vi "Emergency Send To Specific Target.vi"(6 "Paras In":variant, 8 "error in (no error)":errorcluster, 9 "Mail Strategy In":refnum<class "Mail Strategy.lvclass">, 10 "Message In":refnum<class "Message.lvclass">, 11 "Map Tree Queue Messenger in":refnum<class "Map Tree Queue Messenger.lvclass">) -> (0 "error out":errorcluster, 3 "Map Tree Queue Messenger out":refnum<class "Map Tree Queue Messenger.lvclass">)   [LabVIEW 2024, in "Map Tree Queue Messenger.lvclass"]
uses:
  Map Tree Queue Messenger.lvclass
  Ancestor Class/Message/Message.lvclass
  Ancestor Class/Messenger/Mail Strategy/Mail Strategy.lvclass
  Mailman/Simple Tree Queue Mailman/Simple Tree Queue Mailman.lvclass
  Ancestor Class/Messenger/Messenger Map Composite/Messenger Map Composite.lvclass/Messenger Map Composite.ctl
  Mailman/Simple Tree Queue Mailman/Simple Tree Queue Mailman.lvclass/Simple Tree Queue Mailman.ctl
  Map Tree Queue Messenger.lvclass/Map Tree Queue Messenger.ctl
  Mailman/Simple Tree Queue Mailman/Public Data/Write Address Recursive Access.vi
  Ancestor Class/Messenger/Messenger Map Composite/Public Data/Read Child Nodes.vi
  Ancestor Class/Messenger/Messenger/Messenger.lvclass
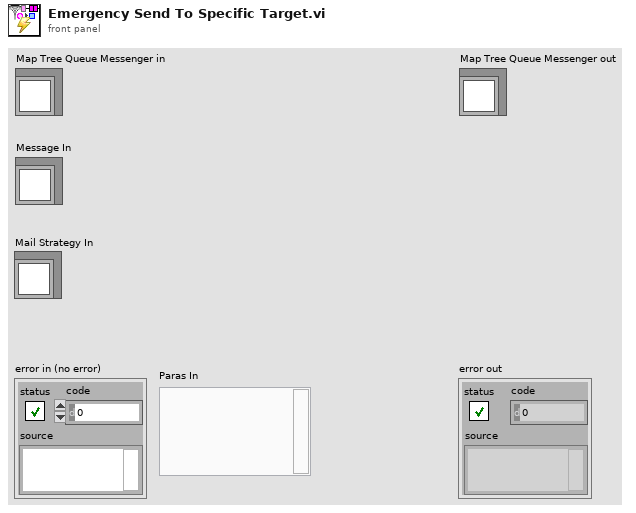
[diagram p1: front panel]
types:
  T1 = typedef "Message Queue.ctl" = refnum<queue>
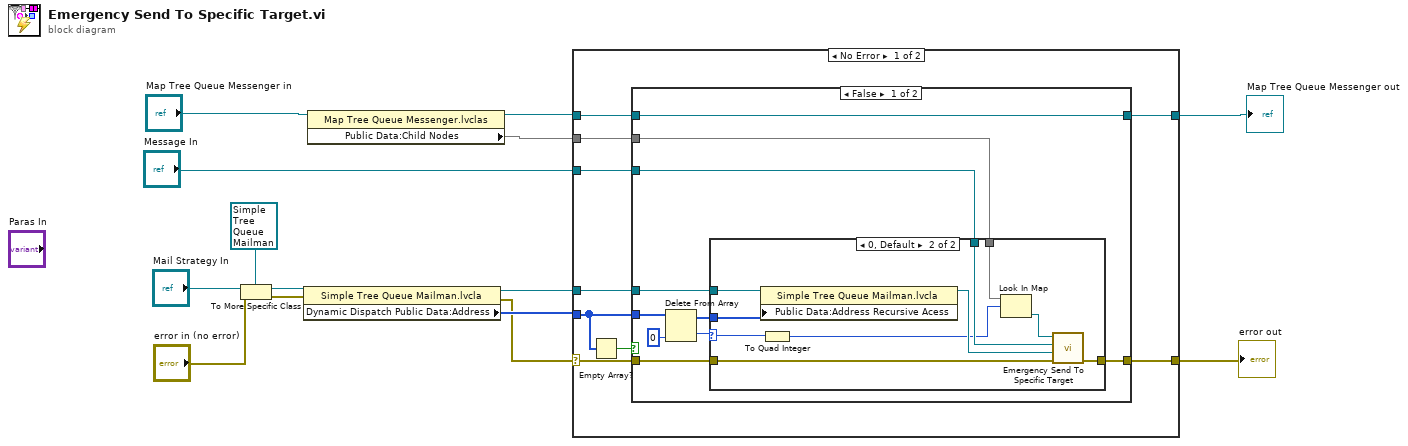
[diagram p0: block diagram]
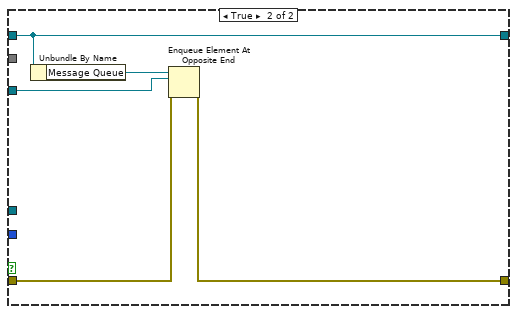
[diagram p3: hidden frame]
diagram:
  n1 = To More Specific Class(target class=refnum<class "Simple Tree Queue Mailman.lvclass"> refnum ("Array Location Mailman.lvclass"), reference="Mail Strategy In", error in="error in (no error)") -> (specific class reference=w12:refnum<class "Simple Tree Queue Mailman.lvclass">, error out=w13:errorcluster)
  n2 = property class="Simple Tree Queue Mailman.lvcla"(reference=w12, error in=w13) -> (reference out=w9:refnum<class "Simple Tree Queue Mailman.lvclass">, error out=w10:errorcluster, "Dynamic Dispatch Public Data:Address"=w11:i32[])
  n3 = property class="Map Tree Queue Messenger.lvclas"(reference="Map Tree Queue Messenger in") -> (reference out=w8:refnum<class "Map Tree Queue Messenger.lvclass">, "Public Data:Child Nodes"=w7:map{i64, refnum<class "Messenger.lvclass">})  [unwired: 1 in, 1 out]
  n4 = case shown="No Error" w10 {
    selector: w10 -> [w18 w50]
    tunnel: w8 -> [w22 w51]
    tunnel: [w20 w51] -> w5
    tunnel: [w17 w50] -> w1
    tunnel: w11 -> [w19 _]
    tunnel: "Message In" -> [w21 _]
    tunnel: w9 -> [w15 _]
    tunnel: w7 -> [w16 _]
    frame No Error {
      n5 = Empty Array?(array=w19) -> (empty?=w23:bool)
      n6 = case shown="False" w23 {
        tunnel: w22 -> [w33 w49]
        tunnel: w21 -> [w30 w47]
        tunnel: [w33 w49] -> w20
        tunnel: w19 -> [w32 _]
        tunnel: w18 -> [w29 w46]
        tunnel: [w28 w45] -> w17
        tunnel: w16 -> [w27 _]
        tunnel: w15 -> [w25 _]
        frame False {
          n7 = Delete From Array(array=w32, index=0) -> (deleted portion=w24:i32, array with subset deleted=w26:i32[])  [unwired: 1 in]
          n8 = case shown="0, Default" w24 {
            selector: w24 -> [_ w36]
            tunnel: w30 -> [_ w44]
            tunnel: w29 -> [w34 w43]
            tunnel: [w34 w42] -> w28
            tunnel: w27 -> [_ w38]
            tunnel: w26 -> [_ w41]
            tunnel: w25 -> [_ w40]
            frame -2147483648..-1 {
            }
            frame 0, Default {
              n9 = property class="Simple Tree Queue Mailman.lvcla"(reference=w40, "Public Data:Address Recursive Acess"=w41) -> (reference out=w39:refnum<class "Simple Tree Queue Mailman.lvclass">)  [unwired: 1 in, 1 out]
              n10 = To Quad Integer(1:w36) -> (0:w35:i64)
              n11 = Look In Map(map=w38, key=w35) -> (value=w37:refnum<class "Messenger.lvclass">)  [unwired: 1 in, 1 out]
              n12 = call-dynamic "Emergency Send To Specific Target.vi"("error in (no error)"=w43, "Mail Strategy In"=w39, "Message In"=w44, "Messenger in"=w37) -> ("error out"=w42:errorcluster)  [unwired: 6 in, 1 out]
            }
          }
        }
        frame True {
          n13 = Unbundle By Name(w49) -> ("Message Queue"=w48:T1)
          n14 = Enqueue Element At Opposite End(queue=w48, element=w47, error in (no error)=w46) -> (error out=w45:errorcluster)  [unwired: 1 in, 2 out]
        }
      }
    }
    frame Error {
    }
  }
  "error out" <- w1
  "Map Tree Queue Messenger out" <- w5
